vi "Read MessageInterface.vi"(11 "Device in":refnum<class "Device.lvclass">) -> (2 "MessageInterface":refnum<class "MessageInterface.lvclass">)   [LabVIEW 2019, in "Device.lvclass"]
uses:
  Device.lvclass
  MessageInterface_class/MessageInterface.lvclass
  Device.lvclass/Device.ctl
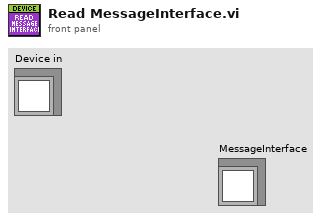
[diagram p1: front panel]
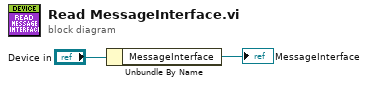
[diagram p0: block diagram]
diagram:
  n1 = Unbundle By Name("Device in") -> ("MessageInterface"=→"MessageInterface":refnum<class "MessageInterface.lvclass">)
